vi "Read Settings.vi"(8 "error in (no error)":errorcluster, 11 "VIStore in":refnum<class "VIStore.lvclass">) -> (0 "error out":errorcluster, 2 "Settings Data":T1, 3 "VIStore out":refnum<class "VIStore.lvclass">)   [LabVIEW 2015, in "VI App Store.lvlib" / "VIStore.lvclass"]
uses:
  VIStore.lvclass
  Classes/Settings Item/Settings Data.ctl
  VIStore.lvclass/VIStore.ctl
  Classes/Settings Item/Settings.lvclass
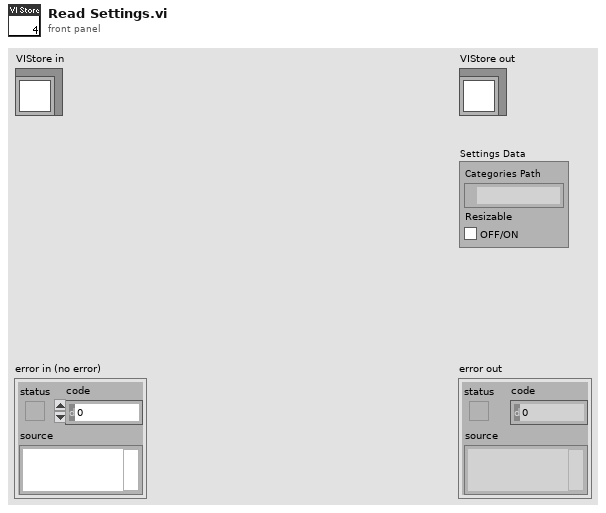
[diagram p1: front panel]
types:
  T1 = typedef "Item Actor.lvlib/Settings.lvclass/Settings Data.ctl" = cluster{"Categories Path":path, "Resizable":bool}
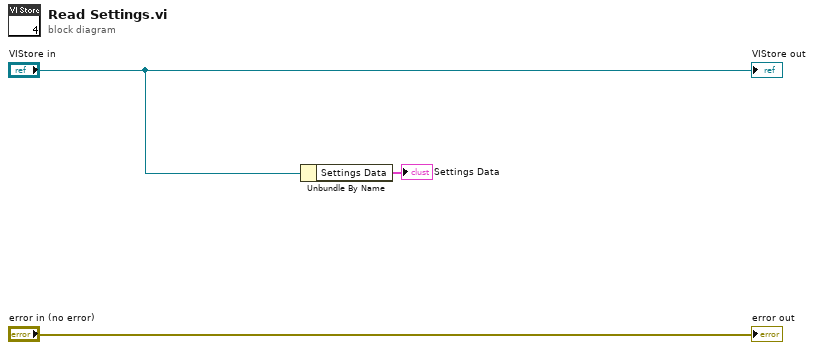
[diagram p0: block diagram]
diagram:
  n1 = Unbundle By Name("VIStore in") -> ("Settings Data"=→"Settings Data":T1)
  "error out" <- "error in (no error)"
  "VIStore out" <- "VIStore in"
